vi "libzmq64 path.vi"() -> (2 "path":path)   [LabVIEW 2019, in "RemoteControl.ZMQ.lvlib" / "libzmq64.lvclass"]
uses:
  libzmq64.lvclass
  <vilib>/addons/zeromq/zeromq.lvlib
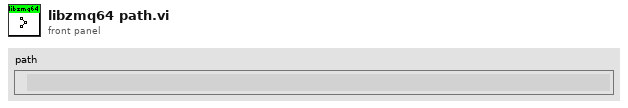
[diagram p1: front panel]
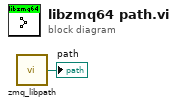
[diagram p0: block diagram]
diagram:
  n1 = call <vilib>:"zmq_libpath.vi"() -> ("path"=→"path":path)
